vi "Derived Data.vi"(8 "error in":errorcluster, 10 "PAS Cell Data in":refnum<class "PAS Cell Data.lvclass">=refnum, 11 "PAS File Obs in":refnum<class "PAS File Obs.lvclass">) -> (0 "error out":errorcluster, 2 "PAS Cell Data Out":refnum<class "PAS Cell Data.lvclass">, 3 "PAS File Obs Out":refnum<class "PAS File Obs.lvclass">)   [LabVIEW 2014, in "PAS File Obs.lvclass"]
uses:
  PAS File Obs.lvclass
  Main/Controls/Cell Data.ctl
  Data/Cell/PAS Cell Data.lvclass
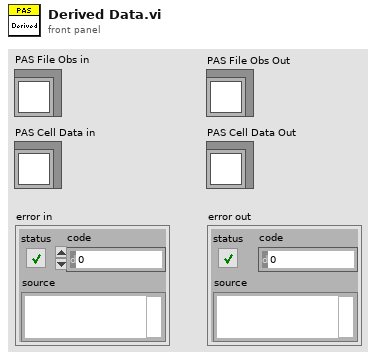
[diagram p1: front panel]
types:
  T1 = typedef "Cell Data.ctl" = u8
  T2 = enum16{"big-endian, network order", "native, host order", "little-endian"}
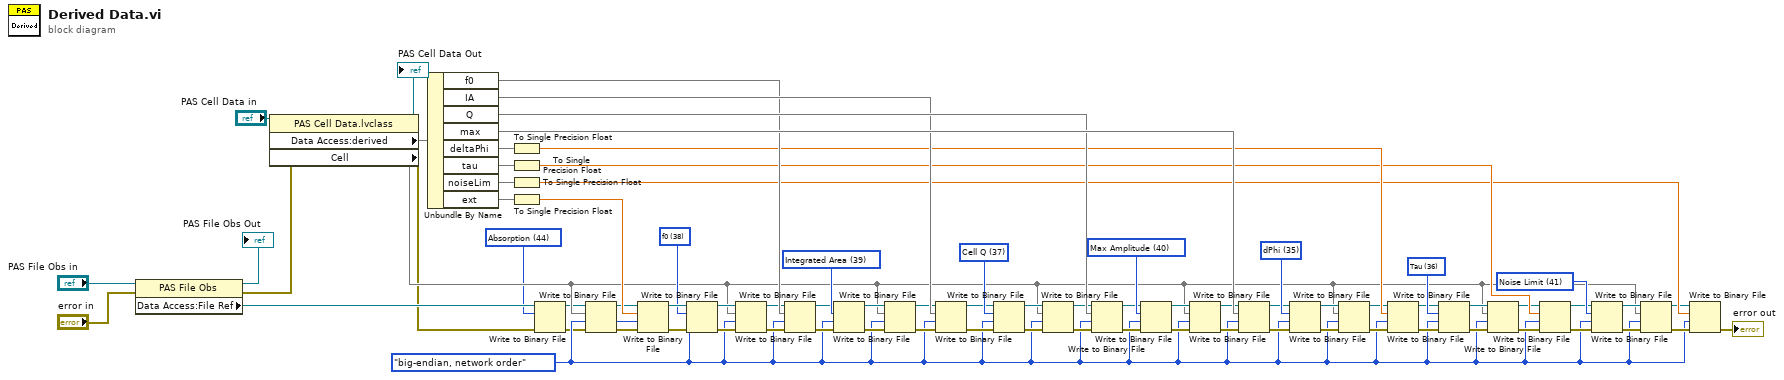
[diagram p0: block diagram]
diagram:
  w59 = T1 41 items=["TEC SP"=23, "TEC Enable"=24, "Qsp"=25, "Tac"=26, "Pac"=27, "Q0ac"=28, "Qac"=29, "Cell TEC T (T1)"=30, "Tmain"=31, "Tv"=32, "RHv"=33, "lasRMS"=34, "dPhi"=35, "Tau"=36, "Cell Q"=37, "f0"=38, "Integrated Area"=39, "Max Amplitude"=40, "Noise Limit"=41, "Lower Noise Bound"=42, "Upper Noise Bound"=43, "Absorption"=44, "fit params"=45, "covariance"=46] ("cellNumData")
  w58 = T1 36 items=["TEC SP"=23, "TEC Enable"=24, "Qsp"=25, "Tac"=26, "Pac"=27, "Q0ac"=28, "Qac"=29, "Cell TEC T (T1)"=30, "Tmain"=31, "Tv"=32, "RHv"=33, "lasRMS"=34, "dPhi"=35, "Tau"=36, "Cell Q"=37, "f0"=38, "Integrated Area"=39, "Max Amplitude"=40, "Noise Limit"=41, "Lower Noise Bound"=42, "Upper Noise Bound"=43, "Absorption"=44, "fit params"=45, "covariance"=46] ("cellNumData")
  w57 = T1 35 items=["TEC SP"=23, "TEC Enable"=24, "Qsp"=25, "Tac"=26, "Pac"=27, "Q0ac"=28, "Qac"=29, "Cell TEC T (T1)"=30, "Tmain"=31, "Tv"=32, "RHv"=33, "lasRMS"=34, "dPhi"=35, "Tau"=36, "Cell Q"=37, "f0"=38, "Integrated Area"=39, "Max Amplitude"=40, "Noise Limit"=41, "Lower Noise Bound"=42, "Upper Noise Bound"=43, "Absorption"=44, "fit params"=45, "covariance"=46] ("cellNumData")
  w56 = T1 40 items=["TEC SP"=23, "TEC Enable"=24, "Qsp"=25, "Tac"=26, "Pac"=27, "Q0ac"=28, "Qac"=29, "Cell TEC T (T1)"=30, "Tmain"=31, "Tv"=32, "RHv"=33, "lasRMS"=34, "dPhi"=35, "Tau"=36, "Cell Q"=37, "f0"=38, "Integrated Area"=39, "Max Amplitude"=40, "Noise Limit"=41, "Lower Noise Bound"=42, "Upper Noise Bound"=43, "Absorption"=44, "fit params"=45, "covariance"=46] ("cellNumData")
  w55 = T1 37 items=["TEC SP"=23, "TEC Enable"=24, "Qsp"=25, "Tac"=26, "Pac"=27, "Q0ac"=28, "Qac"=29, "Cell TEC T (T1)"=30, "Tmain"=31, "Tv"=32, "RHv"=33, "lasRMS"=34, "dPhi"=35, "Tau"=36, "Cell Q"=37, "f0"=38, "Integrated Area"=39, "Max Amplitude"=40, "Noise Limit"=41, "Lower Noise Bound"=42, "Upper Noise Bound"=43, "Absorption"=44, "fit params"=45, "covariance"=46] ("cellNumData")
  w54 = T1 39 items=["TEC SP"=23, "TEC Enable"=24, "Qsp"=25, "Tac"=26, "Pac"=27, "Q0ac"=28, "Qac"=29, "Cell TEC T (T1)"=30, "Tmain"=31, "Tv"=32, "RHv"=33, "lasRMS"=34, "dPhi"=35, "Tau"=36, "Cell Q"=37, "f0"=38, "Integrated Area"=39, "Max Amplitude"=40, "Noise Limit"=41, "Lower Noise Bound"=42, "Upper Noise Bound"=43, "Absorption"=44, "fit params"=45, "covariance"=46] ("cellNumData")
  w53 = T1 38 items=["TEC SP"=23, "TEC Enable"=24, "Qsp"=25, "Tac"=26, "Pac"=27, "Q0ac"=28, "Qac"=29, "Cell TEC T (T1)"=30, "Tmain"=31, "Tv"=32, "RHv"=33, "lasRMS"=34, "dPhi"=35, "Tau"=36, "Cell Q"=37, "f0"=38, "Integrated Area"=39, "Max Amplitude"=40, "Noise Limit"=41, "Lower Noise Bound"=42, "Upper Noise Bound"=43, "Absorption"=44, "fit params"=45, "covariance"=46] ("cellNumData")
  w9 = T2."big-endian, network order" ("byte order (0:big-endian, network order)")
  w5 = T1 44 items=["TEC SP"=23, "TEC Enable"=24, "Qsp"=25, "Tac"=26, "Pac"=27, "Q0ac"=28, "Qac"=29, "Cell TEC T (T1)"=30, "Tmain"=31, "Tv"=32, "RHv"=33, "lasRMS"=34, "dPhi"=35, "Tau"=36, "Cell Q"=37, "f0"=38, "Integrated Area"=39, "Max Amplitude"=40, "Noise Limit"=41, "Lower Noise Bound"=42, "Upper Noise Bound"=43, "Absorption"=44, "fit params"=45, "covariance"=46] ("cellNumData")
  n1 = property class="PAS File Obs"(reference="PAS File Obs in", error in="error in") -> (reference out=→"PAS File Obs Out":refnum<class "PAS File Obs.lvclass">, error out=w4:errorcluster, "Data Access:File Ref"=w8:refnum<file>)
  n2 = property class="PAS Cell Data.lvclass"(reference="PAS Cell Data in", error in=w4) -> (reference out=→"PAS Cell Data Out":refnum<class "PAS Cell Data.lvclass">, error out=w3:errorcluster, "Data Access:derived"=w13, "Cell"=w12)
  n3 = Unbundle By Name(w13) -> ("f0"=w71, "IA"=w72, "Q"=w73, "max"=w74, "deltaPhi"=w75, "tau"=w76, "noiseLim"=w77, "ext"=w78)
  n4 = To Single Precision Float(number=w75) -> (single precision float=w69:sgl)
  n5 = To Single Precision Float(number=w76) -> (single precision float=w68:sgl)
  n6 = To Single Precision Float(number=w77) -> (single precision float=w67:sgl)
  n7 = To Single Precision Float(number=w78) -> (single precision float=w66:sgl)
  n8 = Write to Binary File(file (use dialog)=w8, data=w5, error in=w3) -> (refnum out=w7:refnum<file>, error out=w6:errorcluster)  [unwired: 3 in, 1 out]
  n9 = Write to Binary File(file (use dialog)=w7, data=w12, error in=w6, 9:w9) -> (refnum out=w15:refnum<file>, error out=w16:errorcluster)  [unwired: 2 in, 1 out]
  n10 = Write to Binary File(file (use dialog)=w15, data=w66, error in=w16, 9:w9) -> (refnum out=w64:refnum<file>, error out=w65:errorcluster)  [unwired: 2 in, 1 out]
  n11 = Write to Binary File(file (use dialog)=w64, data=w53, error in=w65, 9:w9) -> (refnum out=w51:refnum<file>, error out=w52:errorcluster)  [unwired: 2 in, 1 out]
  n12 = Write to Binary File(file (use dialog)=w51, data=w12, error in=w52, 9:w9) -> (refnum out=w50:refnum<file>, error out=w49:errorcluster)  [unwired: 2 in, 1 out]
  n13 = Write to Binary File(file (use dialog)=w50, data=w71, error in=w49, 9:w9) -> (refnum out=w48:refnum<file>, error out=w47:errorcluster)  [unwired: 2 in, 1 out]
  n14 = Write to Binary File(file (use dialog)=w48, data=w54, error in=w47, 9:w9) -> (refnum out=w46:refnum<file>, error out=w45:errorcluster)  [unwired: 2 in, 1 out]
  n15 = Write to Binary File(file (use dialog)=w46, data=w12, error in=w45, 9:w9) -> (refnum out=w44:refnum<file>, error out=w43:errorcluster)  [unwired: 2 in, 1 out]
  n16 = Write to Binary File(file (use dialog)=w44, data=w72, error in=w43, 9:w9) -> (refnum out=w42:refnum<file>, error out=w41:errorcluster)  [unwired: 2 in, 1 out]
  n17 = Write to Binary File(file (use dialog)=w42, data=w55, error in=w41, 9:w9) -> (refnum out=w61:refnum<file>, error out=w60:errorcluster)  [unwired: 2 in, 1 out]
  n18 = Write to Binary File(file (use dialog)=w61, data=w12, error in=w60, 9:w9) -> (refnum out=w62:refnum<file>, error out=w63:errorcluster)  [unwired: 2 in, 1 out]
  n19 = Write to Binary File(file (use dialog)=w62, data=w73, error in=w63, 9:w9) -> (refnum out=w40:refnum<file>, error out=w39:errorcluster)  [unwired: 2 in, 1 out]
  n20 = Write to Binary File(file (use dialog)=w40, data=w56, error in=w39, 9:w9) -> (refnum out=w38:refnum<file>, error out=w37:errorcluster)  [unwired: 2 in, 1 out]
  n21 = Write to Binary File(file (use dialog)=w38, data=w12, error in=w37, 9:w9) -> (refnum out=w36:refnum<file>, error out=w35:errorcluster)  [unwired: 2 in, 1 out]
  n22 = Write to Binary File(file (use dialog)=w36, data=w74, error in=w35, 9:w9) -> (refnum out=w34:refnum<file>, error out=w33:errorcluster)  [unwired: 2 in, 1 out]
  n23 = Write to Binary File(file (use dialog)=w34, data=w57, error in=w33, 9:w9) -> (refnum out=w31:refnum<file>, error out=w32:errorcluster)  [unwired: 2 in, 1 out]
  n24 = Write to Binary File(file (use dialog)=w31, data=w12, error in=w32, 9:w9) -> (refnum out=w29:refnum<file>, error out=w30:errorcluster)  [unwired: 2 in, 1 out]
  n25 = Write to Binary File(file (use dialog)=w29, data=w69, error in=w30, 9:w9) -> (refnum out=w27:refnum<file>, error out=w28:errorcluster)  [unwired: 2 in, 1 out]
  n26 = Write to Binary File(file (use dialog)=w27, data=w58, error in=w28, 9:w9) -> (refnum out=w25:refnum<file>, error out=w26:errorcluster)  [unwired: 2 in, 1 out]
  n27 = Write to Binary File(file (use dialog)=w25, data=w12, error in=w26, 9:w9) -> (refnum out=w24:refnum<file>, error out=w23:errorcluster)  [unwired: 2 in, 1 out]
  n28 = Write to Binary File(file (use dialog)=w24, data=w68, error in=w23, 9:w9) -> (refnum out=w22:refnum<file>, error out=w21:errorcluster)  [unwired: 2 in, 1 out]
  n29 = Write to Binary File(file (use dialog)=w22, data=w59, error in=w21, 9:w9) -> (refnum out=w20:refnum<file>, error out=w19:errorcluster)  [unwired: 2 in, 1 out]
  n30 = Write to Binary File(file (use dialog)=w20, data=w12, error in=w19, 9:w9) -> (refnum out=w18:refnum<file>, error out=w17:errorcluster)  [unwired: 2 in, 1 out]
  n31 = Write to Binary File(file (use dialog)=w18, data=w67, error in=w17, 9:w9) -> (error out=→"error out":errorcluster)  [unwired: 2 in, 2 out]
